vi "Keithley DMM6500 DAQ6500 Dual Digitizer for Wide Current Range.vi"() -> ()   [LabVIEW 2020]
doc: "This example shows how to configure dual digitizers and take multiple readings for a wide current range."
uses:
  <instrlib>/Keithley DMM6500 DAQ6500 Series/Keithley DMM6500 DAQ6500 Series.lvlib
panel:
  out "High Range DMM Measurements":sgl[](array[numeric])
  out "Low Range DMM Measurements":sgl[](array[numeric])
  out "Actual Readings":i32
  in  "Shunt Resistor Value (0.001)":sgl=0.001
  in  "Buffer Name High Range DMM (\"digiBuffHigh\")":string="digiBuffHigh"
  in  "Manual Range High Range DMM (10)":dbl=10.0
  in  "VISA Resource Name High Range DMM":refnum<visa-resource-name>
  out "Full Output Data Path":path
  out "Output File Name":string
  in  "Data Extraction Size (100)":i32=100
  in  "Manual Range Low Range DMM (0.1)":dbl=0.1
  in  "Buffer Name Low Range DMM (\"digiBuffLow\")":string="digiBuffLow"
  in  "Count (100000)":u32=100000
  in  "Sample Rate (1E+6)":dbl=1000000.0
  in  "Function (13: Digitize Voltage)":i32(ring)=13 items=["Digitize Voltage"=13, "Digitize Current"=14]
  in  "VISA Resource Name Low Range DMM":refnum<visa-resource-name>
  # "(c) 2019 - 2022 National Instruments.  ALL RIGHTS RESERVED."
  # "INSTRUMENT DEPENDENT SETTINGS"
  # "COMMON SETTINGS"
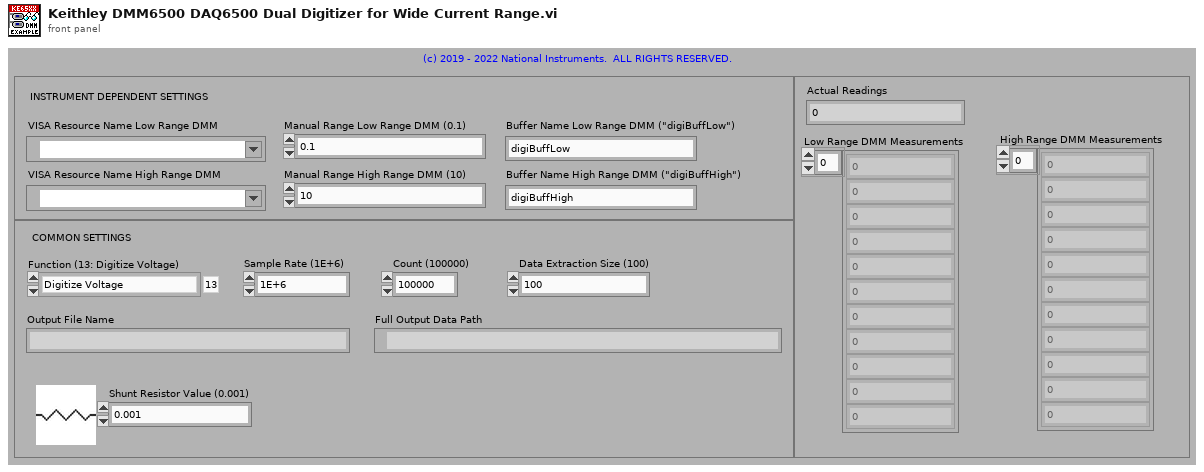
[diagram p1: front panel]
types:
  T1 = enum16{"open", "replace", "create", "open or create", "replace or create", "replace or create with confirmation"}
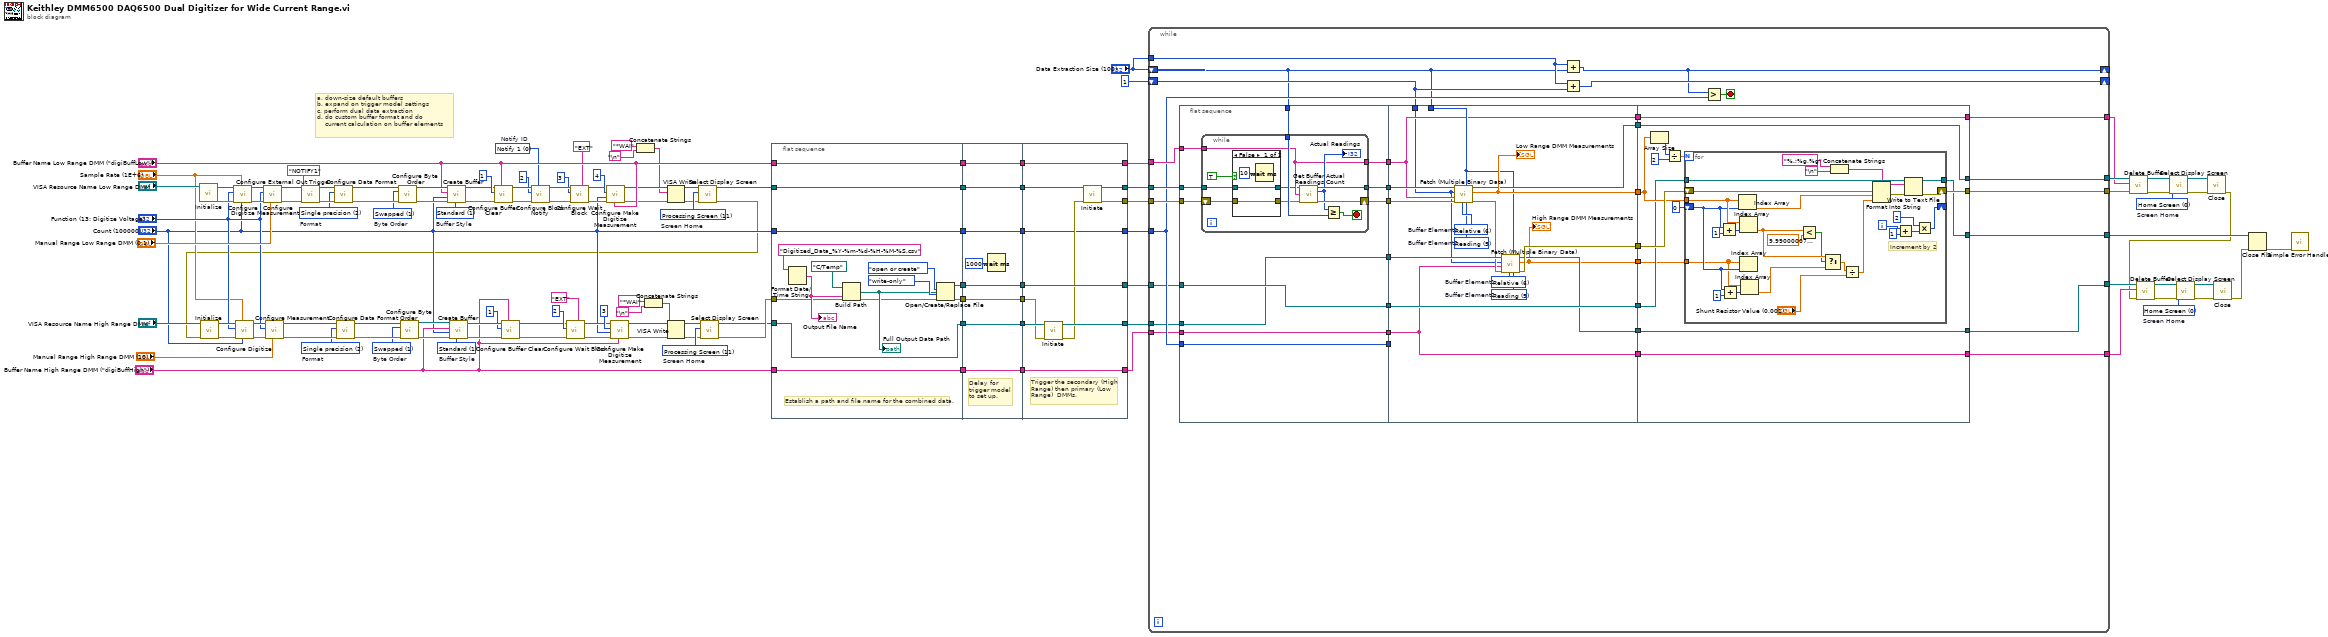
[diagram p0: block diagram]
diagram:
  w11 = u16 0 items=["Home Screen", "Home Large Reading", "Reading Sheet", "Graph Screen", "Histogram", "Functions Swipe", "Graph Swipe", "Secondary Swipe", "Settings Swipe", "Statistics Swipe", "User Swipe", "Processing Screen"]  # Screen Home
  w68 = 0 items=["Notify 1", "Notify 2", "Notify 3", "Notify 4", "Notify 5", "Notify 6", "Notify 7", "Notify 8"]  # Notify ID
  w89 = u16 11 items=["Home Screen", "Home Large Reading", "Reading Sheet", "Graph Screen", "Histogram", "Functions Swipe", "Graph Swipe", "Secondary Swipe", "Settings Swipe", "Statistics Swipe", "User Swipe", "Processing Screen"]  # Screen Home
  w3 = u16 1 items=["Normal", "Swapped"]  # Byte Order
  w4 = u16 2 items=["ASCII", "Double precision", "Single precision"]  # Format
  w96 = 1 items=["Compact", "Standard", "Full", "Writable", "Full Writable"]  # Buffer Style
  w104 = u16 0 items=["Home Screen", "Home Large Reading", "Reading Sheet", "Graph Screen", "Histogram", "Functions Swipe", "Graph Swipe", "Secondary Swipe", "Settings Swipe", "Statistics Swipe", "User Swipe", "Processing Screen"]  # Screen Home
  w109 = u16 11 items=["Home Screen", "Home Large Reading", "Reading Sheet", "Graph Screen", "Histogram", "Functions Swipe", "Graph Swipe", "Secondary Swipe", "Settings Swipe", "Statistics Swipe", "User Swipe", "Processing Screen"]  # Screen Home
  w111 = u16 1 items=["Normal", "Swapped"]  # Byte Order
  w5 = u16 2 items=["ASCII", "Double precision", "Single precision"]  # Format
  w116 = 1 items=["Compact", "Standard", "Full", "Writable", "Full Writable"]  # Buffer Style
  # "a. down-size default buffers\nb. expand on trigger model settings\nc. perform dual data extraction\nd. do custom buffer format and do\n    current calculation on buffer elements"
  n1 = call <instrlib>:"Initialize.vi"("VISA resource name"="VISA Resource Name Low Range DMM") -> ("error out"=w101:errorcluster, "VISA resource name out"=w102:refnum<visa-resource-name>)  [unwired: 9 in]
  n2 = call <instrlib>:"Configure Digitize.vi"("Count (1)"="Count (100000)", "Sample Rate (1E+6)"="Sample Rate (1E+6)", "error in (no error)"=w101, "Function (13: Digitize Voltage)"="Function (13: Digitize Voltage)", "VISA resource name"=w102) -> ("error out"=w122:errorcluster, "VISA resource name out"=w123:refnum<visa-resource-name>)  [unwired: 5 in]
  n3 = call <instrlib>:"Configure Measurement.vi"("Manual Range (1)"="Manual Range Low Range DMM (0.1)", "error in (no error)"=w122, "Function (0: Voltage DC)"="Function (13: Digitize Voltage)", "VISA resource name"=w123) -> ("error out"=w55:errorcluster, "VISA resource name out"=w56:refnum<visa-resource-name>)  [unwired: 6 in]
  n4 = call <instrlib>:"Configure External Out Trigger.vi"("error in (no error)"=w55, "External Stimulus Event (\"NONE\")"="NOTIFY1" ("External Stimulus Event (\"NONE\")"), "VISA resource name"=w56) -> ("error out"=w57:errorcluster, "VISA resource name out"=w58:refnum<visa-resource-name>)  [unwired: 7 in]
  n5 = call <instrlib>:"Configure Data Format.vi"("error in (no error)"=w57, "Format (0: ASCII)"=w5, "VISA resource name"=w58) -> ("error out"=w114:errorcluster, "VISA resource name out"=w115:refnum<visa-resource-name>)  [unwired: 7 in]
  n6 = call <instrlib>:"Configure Byte Order.vi"("VISA resource name"=w115, "Byte Order"=w111, "error in (no error)"=w114) -> ("VISA resource name out"=w113:refnum<visa-resource-name>, "error out"=w112:errorcluster)  [unwired: 11 in]
  n7 = call <instrlib>:"Create Buffer.vi"("Buffer Style (1: Standard)"=w116, "error in (no error)"=w112, "Buffer Size (10)"="Count (100000)", "Buffer Name (\"\")"="Buffer Name Low Range DMM (\"digiBuffLow\")", "VISA resource name"=w113) -> ("error out"=w118:errorcluster, "VISA resource name out"=w117:refnum<visa-resource-name>)  [unwired: 5 in]
  n8 = call <instrlib>:"Configure Buffer Clear.vi"("Buffer Name (\"\")"="Buffer Name Low Range DMM (\"digiBuffLow\")", "error in (no error)"=w118, "Block Number (1)"=u32 1 ("Block Number (0)"), "VISA resource name"=w117) -> ("error out"=w70:errorcluster, "VISA resource name out"=w71:refnum<visa-resource-name>)  [unwired: 6 in]
  n9 = call <instrlib>:"Configure Block Notify.vi"("Notify ID (0: Notify 1)"=w68, "error in (no error)"=w70, "Block Number (1)"=u32 2 ("Block Number (0)"), "VISA resource name"=w71) -> ("error out"=w75:errorcluster, "VISA resource name out"=w74:refnum<visa-resource-name>)  [unwired: 6 in]
  n10 = call <instrlib>:"Configure Wait Block.vi"("Event1 (\"\")"="EXT" ("Event1 (\"\")"), "error in (no error)"=w75, "Block Number (1)"=u32 3 ("Block Number (0)"), "VISA resource name"=w74) -> ("error out"=w66:errorcluster, "VISA resource name out"=w67:refnum<visa-resource-name>)  [unwired: 6 in]
  n11 = call <instrlib>:"Configure Make Digitize Measurement.vi"("Buffer Name (\"defbuffer1\")"="Buffer Name Low Range DMM (\"digiBuffLow\")", "error in (no error)"=w66, "Readings Count (1)"="Count (100000)", "Block Number (1)"=u32 4 ("Block Number (0)"), "VISA resource name"=w67) -> ("error out"=w32:errorcluster, "VISA resource name out"=w33:refnum<visa-resource-name>)  [unwired: 5 in]
  n12 = Concatenate Strings("*WAI" ("string"), "\n") -> (w29:string)
  n13 = Concatenate Strings("*WAI" ("string"), "\n") -> (w76:string)
  n14 = VISA Write(VISA resource name=w33, write buffer=w29, error in (no error)=w32) -> (VISA resource name out=w30:refnum<visa-resource-name>, error out=w31:errorcluster)  [unwired: 1 out]
  n15 = call <instrlib>:"Select Display Screen.vi"("error in (no error)"=w31, "Screen Home"=w109, "VISA resource name"=w30) -> ("error out"=w1:errorcluster, "VISA resource name out"=w81:refnum<visa-resource-name>)  [unwired: 7 in]
  n16 = call <instrlib>:"Initialize.vi"("error in (no error)"=w1, "VISA resource name"="VISA Resource Name High Range DMM") -> ("error out"=w87:errorcluster, "VISA resource name out"=w88:refnum<visa-resource-name>)  [unwired: 8 in]
  n17 = call <instrlib>:"Configure Digitize.vi"("Count (1)"="Count (100000)", "Sample Rate (1E+6)"="Sample Rate (1E+6)", "error in (no error)"=w87, "Function (13: Digitize Voltage)"="Function (13: Digitize Voltage)", "VISA resource name"=w88) -> ("error out"=w99:errorcluster, "VISA resource name out"=w100:refnum<visa-resource-name>)  [unwired: 5 in]
  n18 = call <instrlib>:"Configure Measurement.vi"("Manual Range (1)"="Manual Range High Range DMM (10)", "error in (no error)"=w99, "Function (0: Voltage DC)"="Function (13: Digitize Voltage)", "VISA resource name"=w100) -> ("error out"=w94:errorcluster, "VISA resource name out"=w95:refnum<visa-resource-name>)  [unwired: 6 in]
  n19 = call <instrlib>:"Configure Data Format.vi"("error in (no error)"=w94, "Format (0: ASCII)"=w4, "VISA resource name"=w95) -> ("error out"=w92:errorcluster, "VISA resource name out"=w93:refnum<visa-resource-name>)  [unwired: 7 in]
  n20 = call <instrlib>:"Configure Byte Order.vi"("VISA resource name"=w93, "Byte Order"=w3, "error in (no error)"=w92) -> ("VISA resource name out"=w91:refnum<visa-resource-name>, "error out"=w90:errorcluster)  [unwired: 11 in]
  n21 = call <instrlib>:"Create Buffer.vi"("Buffer Style (1: Standard)"=w96, "error in (no error)"=w90, "Buffer Size (10)"="Count (100000)", "Buffer Name (\"\")"="Buffer Name High Range DMM (\"digiBuffHigh\")", "VISA resource name"=w91) -> ("error out"=w98:errorcluster, "VISA resource name out"=w97:refnum<visa-resource-name>)  [unwired: 5 in]
  n22 = call <instrlib>:"Configure Buffer Clear.vi"("Buffer Name (\"\")"="Buffer Name High Range DMM (\"digiBuffHigh\")", "error in (no error)"=w98, "Block Number (1)"=u32 1 ("Block Number (0)"), "VISA resource name"=w97) -> ("error out"=w62:errorcluster, "VISA resource name out"=w63:refnum<visa-resource-name>)  [unwired: 6 in]
  n23 = call <instrlib>:"Configure Wait Block.vi"("Event1 (\"\")"="EXT" ("Event1 (\"\")"), "error in (no error)"=w62, "Block Number (1)"=u32 2 ("Block Number (0)"), "VISA resource name"=w63) -> ("error out"=w60:errorcluster, "VISA resource name out"=w61:refnum<visa-resource-name>)  [unwired: 6 in]
  n24 = call <instrlib>:"Configure Make Digitize Measurement.vi"("Buffer Name (\"defbuffer1\")"="Buffer Name High Range DMM (\"digiBuffHigh\")", "error in (no error)"=w60, "Readings Count (1)"="Count (100000)", "Block Number (1)"=u32 3 ("Block Number (0)"), "VISA resource name"=w61) -> ("error out"=w39:errorcluster, "VISA resource name out"=w40:refnum<visa-resource-name>)  [unwired: 5 in]
  n25 = VISA Write(VISA resource name=w40, write buffer=w76, error in (no error)=w39) -> (VISA resource name out=w37:refnum<visa-resource-name>, error out=w38:errorcluster)  [unwired: 1 out]
  n26 = call <instrlib>:"Select Display Screen.vi"("error in (no error)"=w38, "Screen Home"=w89, "VISA resource name"=w37) -> ("error out"=w82:errorcluster, "VISA resource name out"=w80:refnum<visa-resource-name>)  [unwired: 7 in]
  n27 = flat-sequence {
    tunnel: w82 -> [w131]
    tunnel: w81 -> [w129]
    tunnel: w80 -> [w128]
    tunnel: [w132] -> w54
    tunnel: [w130] -> w52
    tunnel: [w129] -> w50
    tunnel: [w128] -> w48
    tunnel: "Buffer Name Low Range DMM (\"digiBuffLow\")" -> [w127]
    tunnel: [w127] -> w46
    tunnel: "Buffer Name High Range DMM (\"digiBuffHigh\")" -> [w126]
    tunnel: [w126] -> w44
    tunnel: "Count (100000)" -> [w125]
    tunnel: [w125] -> w42
    tunnel: w54 -> [w146]
    tunnel: [w146] -> w53
    tunnel: w52 -> [w145]
    tunnel: [w145] -> w51
    tunnel: w50 -> [w144]
    tunnel: [w144] -> w49
    tunnel: w48 -> [w143]
    tunnel: [w143] -> w47
    tunnel: w46 -> [w142]
    tunnel: [w142] -> w45
    tunnel: w44 -> [w141]
    tunnel: [w141] -> w43
    tunnel: w42 -> [w140]
    tunnel: [w140] -> w41
    tunnel: [w157] -> w24
    tunnel: w53 -> [w157]
    tunnel: w51 -> [w153]
    tunnel: w49 -> [w152]
    tunnel: w47 -> [w155]
    tunnel: [w156] -> w23
    tunnel: w45 -> [w156]
    tunnel: [w154] -> w18
    tunnel: [w151] -> w27
    tunnel: [w149] -> w26
    tunnel: w43 -> [w148]
    tunnel: [w148] -> w16
    tunnel: [w147] -> w25
    tunnel: w41 -> [w147]
    frame #0 {
      # "Establish a path and file name for the combined data."
      n28 = Format Date/Time String(time format string (%c)="Digitized_Data_%Y-%m-%d-%H-%M-%S.csv") -> (date/time string=w138:string)  [unwired: 2 in]
      "Output File Name" <- w138
      n29 = Build Path(base path=path "C:/Temp" ("file path (use dialog)"), name or relative path=w138) -> (appended path=w133:path)
      "Full Output Data Path" <- w133
      n30 = Open/Create/Replace File(file path (use dialog)=w133, error in=w131, operation (0:open)=T1."open or create", access (0:read/write)=enum16{"read/write", "read-only", "write-only"}."write-only") -> (refnum out=w132:refnum<file>, error out=w130:errorcluster)  [unwired: 2 in, 1 out]
    }
    frame #1 {
      # "Delay for \ntrigger model\nto set up."
      n31 = Wait (ms)(milliseconds to wait=u32 1000) -> ()  [unwired: 1 out]
    }
    frame #2 {
      # "Trigger the secondary (High\nRange) then primary (Low\nRange)  DMMs."
      n32 = call <instrlib>:"Initiate.vi"("error in (no error)"=w153, "VISA resource name"=w155) -> ("error out"=w150:errorcluster, "VISA resource name out"=w154:refnum<visa-resource-name>)  [unwired: 8 in]
      n33 = call <instrlib>:"Initiate.vi"("error in (no error)"=w150, "VISA resource name"=w152) -> ("error out"=w149:errorcluster, "VISA resource name out"=w151:refnum<visa-resource-name>)  [unwired: 8 in]
    }
  }
  n34 = while {
    shift-right: [w191] -> _
    shift-left: 1 ("Start Index (1)") -> [w177]
    shift-right: [w189] -> _
    shift-left: "Data Extraction Size (100)" -> [w176]
    tunnel: "Data Extraction Size (100)" -> [w188]
    tunnel: w27 -> [w186]
    tunnel: w26 -> [w185]
    tunnel: w23 -> [w187]
    tunnel: [w175] -> w22
    tunnel: [w165] -> w21
    tunnel: w25 -> [w184]
    tunnel: w24 -> [w183]
    tunnel: [w164] -> w19
    tunnel: w18 -> [w169]
    tunnel: [w163] -> w17
    tunnel: w16 -> [w162]
    tunnel: [w159] -> w10
    tunnel: [w158] -> w9
    stop <- w190 stop-if-true
    n35 = flat-sequence {
      tunnel: w187 -> [w202]
      tunnel: w186 -> [w201]
      tunnel: w185 -> [w200]
      tunnel: w176 -> [w196]
      tunnel: w184 -> [w195]
      tunnel: w183 -> [w194]
      tunnel: [w199] -> w182
      tunnel: [w198] -> w181
      tunnel: [w197] -> w180
      tunnel: [w195] -> w179
      tunnel: [w194] -> w178
      tunnel: w169 -> [w193]
      tunnel: [w193] -> w168
      tunnel: w162 -> [w192]
      tunnel: [w192] -> w161
      tunnel: w182 -> [w220]
      tunnel: w181 -> [w233]
      tunnel: w180 -> [w232]
      tunnel: w179 -> [_]
      tunnel: w178 -> [w236]
      tunnel: w177 -> [w219]
      tunnel: w176 -> [w227]
      tunnel: [w220] -> w174
      tunnel: [w236] -> w173
      tunnel: [w231] -> w172
      tunnel: [w230] -> w171
      tunnel: [w225] -> w170
      tunnel: w168 -> [w228]
      tunnel: [w224] -> w167
      tunnel: [w222] -> w166
      tunnel: w161 -> [w221]
      tunnel: [w221] -> w160
      tunnel: [w249] -> w175
      tunnel: [w250] -> w163
      tunnel: w174 -> [w250]
      tunnel: w173 -> [w242]
      tunnel: w172 -> [w243]
      tunnel: w171 -> [w249]
      tunnel: w170 -> [w244]
      tunnel: w167 -> [w237]
      tunnel: w166 -> [w241]
      tunnel: [w240] -> w165
      tunnel: [w239] -> w164
      tunnel: w160 -> [w238]
      tunnel: [w238] -> w158
      tunnel: [w237] -> w159
      frame #0 {
        n36 = while {
          tunnel: w202 -> [w208]
          shift-right: [w212] -> w197
          shift-left: w200 -> [w207]
          tunnel: w196 -> [w209]
          tunnel: w201 -> [w205]
          tunnel: [w213] -> w198
          tunnel: [w208] -> w199
          stop <- w211 stop-if-true
          n37 = case shown="False" TRUE {
            tunnel: w207 -> [w215 w218]
            tunnel: [w215 w218] -> w206
            tunnel: w205 -> [w216 w217]
            tunnel: [w216 w217] -> w204
            frame False {
              n38 = Wait (ms)(milliseconds to wait=u32 10) -> ()  [unwired: 1 out]
            }
            frame True {
            }
          }
          n39 = call <instrlib>:"Get Buffer Actual Readings Count.vi"("VISA resource name"=w204, "Buffer Name (defbuffer1)"=w208, "error in (no error)"=w206) -> ("VISA resource name out"=w213:refnum<visa-resource-name>, "Actual Readings"=w210:i32, "error out"=w212:errorcluster)  [unwired: 10 in]
          "Actual Readings" <- w210
          n40 = Greater Or Equal?(x=w210, y=w209) -> (x >= y?=w211:bool)
        }
      }
      frame #1 {
        w223 = 5 items=["", "Date", "Extra", "Formatted", "Fractional", "Reading", "Relative", "Seconds", "Status", "Time", "Tstamp", "Unit", "CHAN", "Extra Form", "Extra Unit"]  # Buffer Element2
        w229 = 6 items=["", "Date", "Extra", "Formatted", "Fractional", "Reading", "Relative", "Seconds", "Status", "Time", "Tstamp", "Unit", "CHAN", "Extra Format", "Extra Unit"]  # Buffer Element1
        w234 = 5 items=["", "Date", "Extra", "Formatted", "Fractional", "Reading", "Relative", "Seconds", "Status", "Time", "Tstamp", "Unit", "CHAN", "Extra Form", "Extra Unit"]  # Buffer Element2
        w235 = 6 items=["", "Date", "Extra", "Formatted", "Fractional", "Reading", "Relative", "Seconds", "Status", "Time", "Tstamp", "Unit", "CHAN", "Extra Format", "Extra Unit"]  # Buffer Element1
        n41 = call <instrlib>:"Fetch (Multiple Binary Data).vi"("Buffer Element2"=w234, "End Index (10)"=w227, "Buffer Element1"=w235, "error in (no error)"=w232, "Buffer Name"=w220, "Start Index (1)"=w219, "VISA resource name"=w233) -> ("error out"=w226:errorcluster, "Measurements"=w231:sgl[], "VISA resource name out"=w230:refnum<visa-resource-name>)  [unwired: 2 in]
        "Low Range DMM Measurements" <- w231
        n42 = call <instrlib>:"Fetch (Multiple Binary Data).vi"("Buffer Element2"=w223, "End Index (10)"=w227, "Buffer Element1"=w229, "error in (no error)"=w226, "Buffer Name"=w221, "Start Index (1)"=w219, "VISA resource name"=w228) -> ("error out"=w225:errorcluster, "Measurements"=w222:sgl[], "VISA resource name out"=w224:refnum<visa-resource-name>)  [unwired: 2 in]
        "High Range DMM Measurements" <- w222
      }
      frame #2 {
        n43 = Array Size(array=w243) -> (size(s)=w247:i32)
        n44 = Divide(x=w247, y=2 ("x")) -> (x/y=w245:dbl)
        n45 = for {
          N: w245 -> [_]
          shift-right: [w272] -> w240
          shift-left: w244 -> [w273]
          tunnel: w243 -> [w271]
          tunnel: w242 -> [w279]
          tunnel: [w278] -> w239
          shift-right: [w264] -> _
          shift-left: 0 ("index") -> [w260]
          tunnel: w241 -> [w259]
          i -> [w265]
          # "Increment by 2"
          n46 = Add(x=w260, y=1) -> (x+y=w268:i32)
          n47 = Add(x=w260, y=1) -> (x+y=w261:i32)
          n48 = Index Array(array=w271, index=w260) -> (element=w270:sgl)
          n49 = Index Array(array=w271, index=w268) -> (element=w257:sgl)
          n50 = Index Array(array=w259, index=w260) -> ()  [unwired: 1 out]
          n51 = Index Array(array=w259, index=w261) -> (element=w258:sgl)
          n52 = Less?(x=w257, y=sgl 9.99e+36) -> (x < y?=w256:bool)
          n53 = Select(t=w257, s=w256, f=w258) -> (s? t:f=w253:sgl)
          n54 = Concatenate Strings("%.;%g,%g" ("format string"), "\n") -> (w274:string)
          n55 = Divide(x=w253, y="Shunt Resistor Value (0.001)") -> (x/y=w252:sgl)
          n56 = Format Into String(format string=w274, error in=w273, w270, w252) -> (resulting string=w263:string, error out=w277:errorcluster)  [unwired: 1 in]
          n57 = Add(x=w265, y=1) -> (x+y=w266:i32)
          n58 = Write to Text File(file (use dialog)=w279, text=w263, error in=w277) -> (refnum out=w278:refnum<file>, error out=w272:errorcluster)  [unwired: 1 in, 1 out]
          n59 = Multiply(x=2, y=w266) -> (x*y=w264:i32)
        }
      }
    }
    n60 = Add(x=w188, y=w176) -> (x+y=w189:i32)
    n61 = Add(x=w188, y=w177) -> (x+y=w191:i32)
    n62 = Greater?(x=w189, y=w184) -> (0:w190:bool)
  }
  n63 = call <instrlib>:"Delete Buffer.vi"("error in (no error)"=w21, "Buffer Name (\"\")"=w17, "VISA resource name"=w22) -> ("error out"=w107:errorcluster, "VISA resource name out"=w108:refnum<visa-resource-name>)  [unwired: 7 in]
  n64 = call <instrlib>:"Select Display Screen.vi"("error in (no error)"=w107, "Screen Home"=w104, "VISA resource name"=w108) -> ("error out"=w106:errorcluster, "VISA resource name out"=w105:refnum<visa-resource-name>)  [unwired: 7 in]
  n65 = call <instrlib>:"Close.vi"("error in (no error)"=w106, "VISA resource name"=w105) -> ("error out"=w8:errorcluster)  [unwired: 9 in]
  n66 = call <instrlib>:"Delete Buffer.vi"("error in (no error)"=w8, "Buffer Name (\"\")"=w9, "VISA resource name"=w10) -> ("error out"=w14:errorcluster, "VISA resource name out"=w15:refnum<visa-resource-name>)  [unwired: 7 in]
  n67 = call <instrlib>:"Select Display Screen.vi"("error in (no error)"=w14, "Screen Home"=w11, "VISA resource name"=w15) -> ("error out"=w13:errorcluster, "VISA resource name out"=w12:refnum<visa-resource-name>)  [unwired: 7 in]
  n68 = call <instrlib>:"Close.vi"("error in (no error)"=w13, "VISA resource name"=w12) -> ("error out"=w7:errorcluster)  [unwired: 9 in]
  n69 = Close File(refnum=w19, error in=w7) -> (error out=w110:errorcluster)  [unwired: 1 out]
  n70 = call <vilib>:"Simple Error Handler.vi"("error in (no error)"=w110) -> ()  [unwired: 4 in, 5 out]
